vi "PAINEL DE TESTES 2808.vi"() -> ()   [LabVIEW 2017]
panel:
  out "ADDR NÃO COMPATÍVEL":bool
  in  "ME":bool
  in  "HMP":bool
  in  "SMP":bool
  out "TAM_P":bool
  out "POS_1":bool
  out "MAT":bool
  out "POS_2":bool
  out "COR_3":bool
  out "PDS":bool
  out "COR_2":bool
  out "PEE":bool
  out "POS_4":bool
  out "COR_1":bool
  out "POS_3":bool
  out "TAM_M":bool
  out "TAM_G":bool
  out "ADDR 100":bool
  out "ADDR 101":bool
  out "ADDR 011":bool
  out "ADDR 010":bool
  in  "Array":bool[](array[boolean])
  out "INPUT ARRAYS":bool[](array[boolean])
  in  "time stamp":timestamp format="%<%X\n%x>T"
  # "UNIVERSIDADE FEDERAL DE SÃO JOÃO DEL-REI"
  # "CAMPUS ALTO PARAOPEBA - ENGENHARIA MECATRÔNICA\nLABORATÓRIO DE CONTROLE E AUTOMAÇÃO"
  # "PAINEL DE TESTES DO MÓDULO 2808"
  # "P1.0"
  # "P1.1"
  # "P1.2"
  # "D0"
  # "D1"
  # "D2"
  # "D3"
  # "D4"
  # "D5"
  # "D6"
  # "D7"
  # "ADDR 010"
  # "TAGS:\nPEE - PEÇA NA ENTRADA DA ESTEIRA\nMAT - MATERIAL DA PEÇA (T=METAL)\nCOR_1 - PEÇA DA COR 1\nCOR_2 - PEÇA DA COR 2\nCOR_3 - PEÇA DA COR 3\nTAM_G - PEÇA GRANDE\nTAM_M - PEÇA MÉDIA\nTAM_P - PEÇA PEQUENA\nPOS_1 - HASTE NA POSIÇÃO 1\nPOS_2 - HASTE NA POSIÇÃO 2\nPOS_3 - HASTE NA POSIÇÃO 3\nPOS_4 - HASTE NA POSIÇÃO 4\nPDS - PEÇA DEPOSITADA NO SLOT\n\nSMP - SENTIDO DO MOTOR DE PASSO\nHMP - HABILITA MOTOR DE PASSO\nME - MOTOR ESTEIRA"
  # "ADDR 011"
  # "ENCODER"
  # "ADDR 101"
  # "ADDR 100"
  # "TAM_G"
  # "TAM_P"
  # "TAM_M"
  # "SMP"
  # "POS_1"
  # "POS_2"
  # "POS_3"
  # "POS_4"
  # "PEE"
  # "MAT"
  # "COR_1,2,3"
  # "HMP"
  # "ME"
  # "PDS"
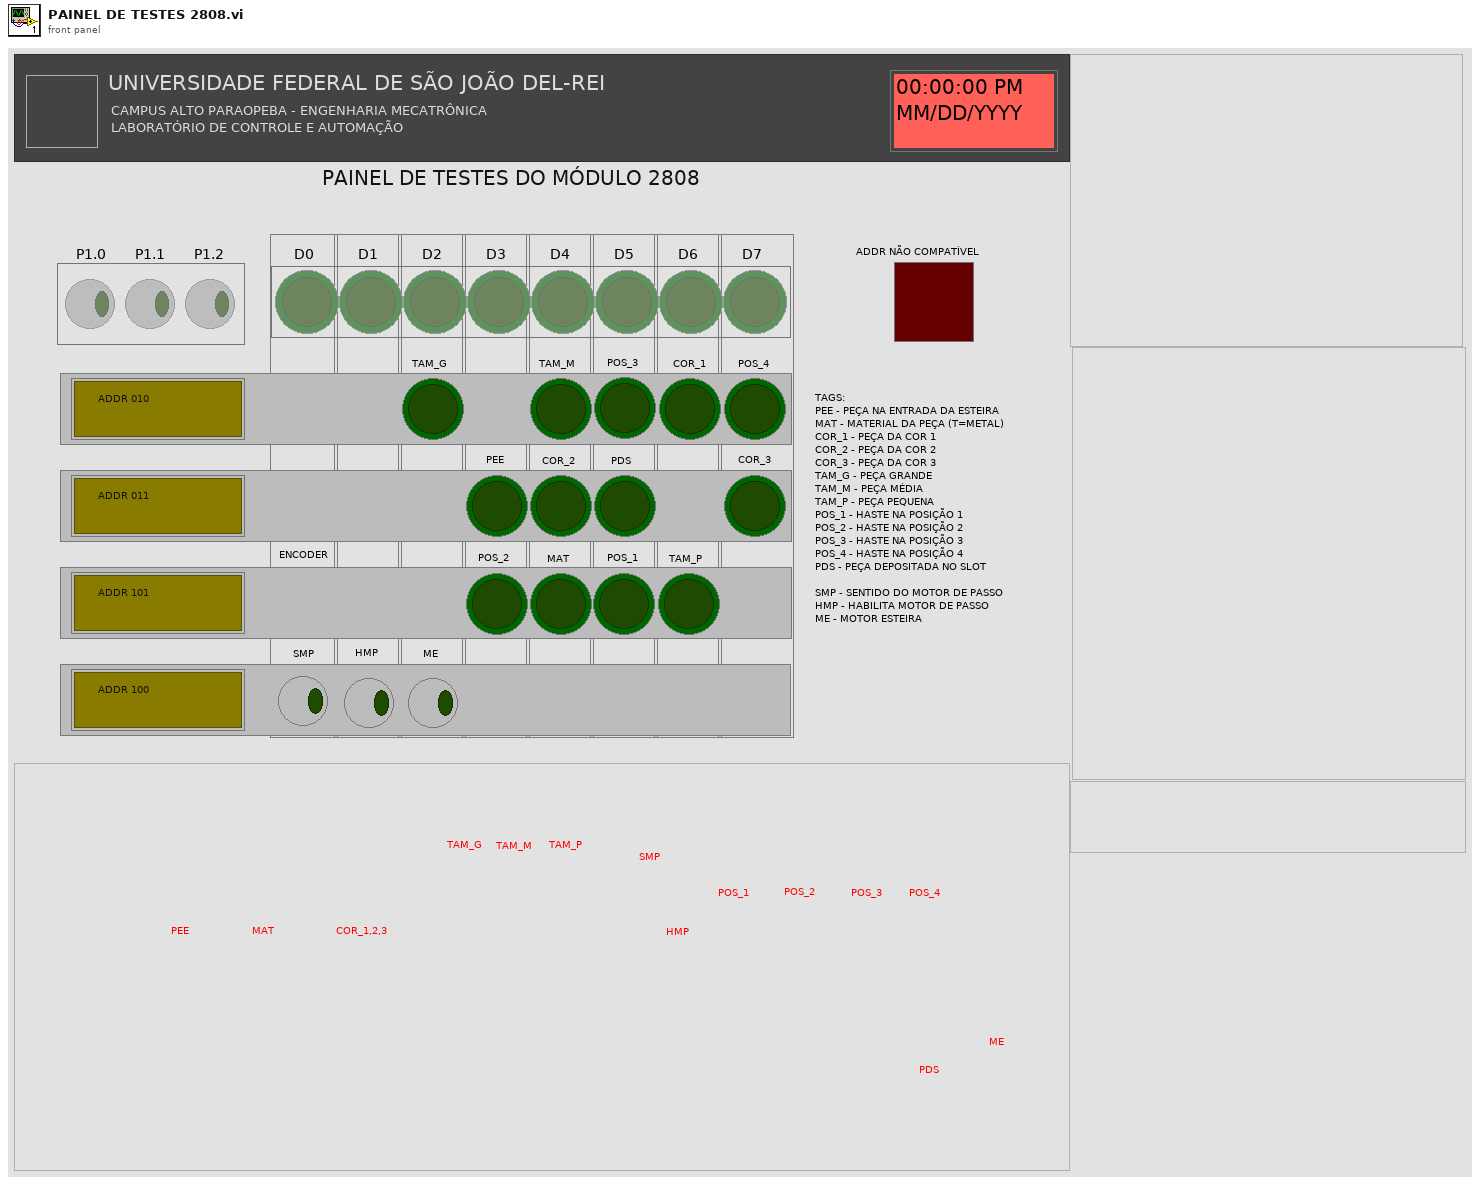
[diagram p1: front panel]
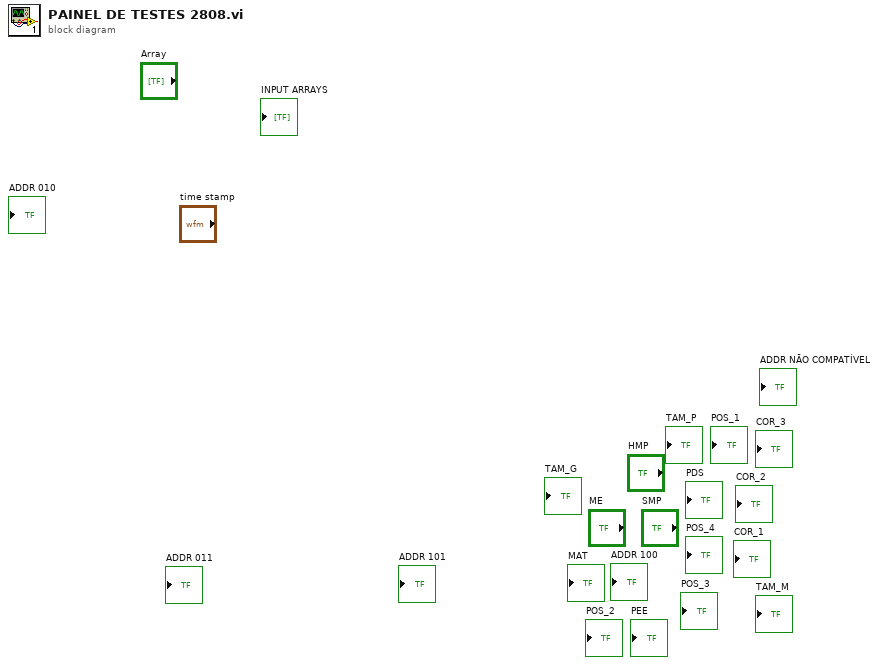
[diagram p0: block diagram]
diagram:
